vi "onAddHeaders.vi"(8 "error in (no error)":errorcluster, 10 "headers":cluster{"header":string, "value":string}[](array[cluster]), 11 "httpHeaders in":refnum<class "httpHeaders.lvclass">) -> (0 "error out":errorcluster, 3 "httpHeaders out":refnum<class "httpHeaders.lvclass">)   [LabVIEW 2020, in "httpClient.lvlib" / "httpHeaders.lvclass"]
uses:
  httpHeaders.lvclass
  httpHeaders.lvclass/httpHeaders.ctl
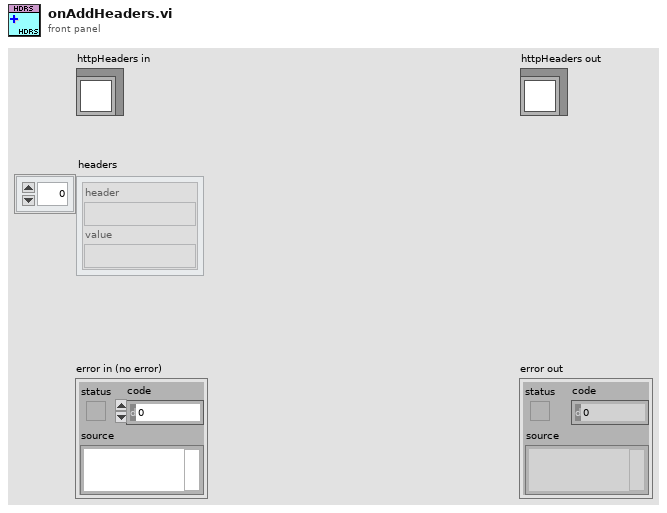
[diagram p1: front panel]
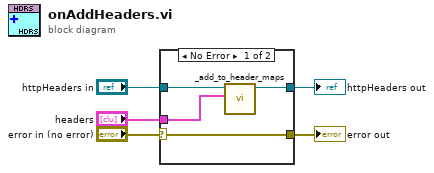
[diagram p0: block diagram]
diagram:
  n1 = case shown="No Error" "error in (no error)" {
    selector: "error in (no error)" -> [w9 w11]
    tunnel: [w9 w11] -> w4
    tunnel: [w8 w10] -> w2
    tunnel: "httpHeaders in" -> [w7 w10]
    tunnel: "headers" -> [w6 _]
    frame No Error {
      n2 = call "_add_to_header_maps.vi"("ordered headers"=w6, "httpHeaders in"=w7) -> ("httpHeaders out"=w8:refnum<class "httpHeaders.lvclass">)  [unwired: 9 in]
    }
    frame Error {
    }
  }
  "error out" <- w4
  "httpHeaders out" <- w2
